vi "获取参数解析.vi"(11 "输入字符串":string) -> (3 "获取参数(定点数)":T1)   [LabVIEW 2016, in "环境动力监测库.lvlib" / "空调库.lvlib"]
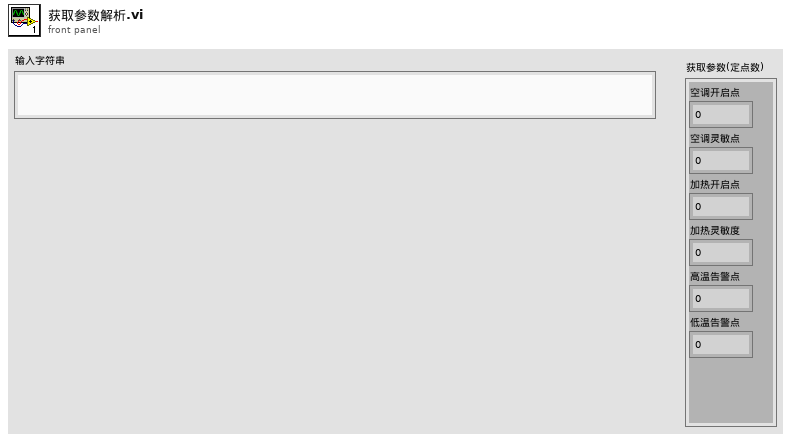
[diagram p1: front panel]
types:
  T1 = cluster{"空调开启点":u16, "空调灵敏点":u16, "加热开启点":u16, "加热灵敏度":u16, "高温告警点":u16, "低温告警点":u16}
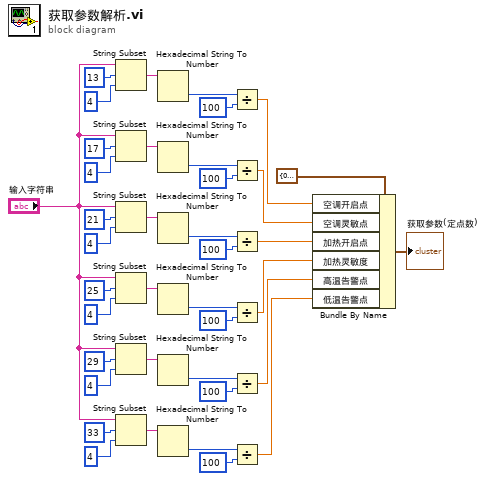
[diagram p0: block diagram]
diagram:
  n1 = String Subset(string="输入字符串", offset (0)=13 ("偏移量(0)"), length (rest)=4 ("长度（剩余）")) -> (substring=w37:string)
  n2 = String Subset(string="输入字符串", offset (0)=17 ("偏移量(0)"), length (rest)=4 ("长度（剩余）")) -> (substring=w34:string)
  n3 = String Subset(string="输入字符串", offset (0)=21 ("偏移量(0)"), length (rest)=4 ("长度（剩余）")) -> (substring=w33:string)
  n4 = String Subset(string="输入字符串", offset (0)=25 ("偏移量(0)"), length (rest)=4 ("长度（剩余）")) -> (substring=w28:string)
  n5 = String Subset(string="输入字符串", offset (0)=29 ("偏移量(0)"), length (rest)=4 ("长度（剩余）")) -> (substring=w20:string)
  n6 = String Subset(string="输入字符串", offset (0)=33 ("偏移量(0)"), length (rest)=4 ("长度（剩余）")) -> (substring=w25:string)
  n7 = Hexadecimal String To Number(string=w37) -> (number=w18:u32)  [unwired: 2 in, 1 out]
  n8 = Hexadecimal String To Number(string=w34) -> (number=w14:u32)  [unwired: 2 in, 1 out]
  n9 = Hexadecimal String To Number(string=w33) -> (number=w9:u32)  [unwired: 2 in, 1 out]
  n10 = Hexadecimal String To Number(string=w28) -> (number=w7:u32)  [unwired: 2 in, 1 out]
  n11 = Hexadecimal String To Number(string=w20) -> (number=w6:u32)  [unwired: 2 in, 1 out]
  n12 = Hexadecimal String To Number(string=w25) -> (number=w2:u32)  [unwired: 2 in, 1 out]
  n13 = Divide(x=w18, y=u32 100) -> (x/y=w16:dbl)
  n14 = Divide(x=w14, y=u32 100) -> (x/y=w13:dbl)
  n15 = Divide(x=w9, y=u32 100) -> (x/y=w8:dbl)
  n16 = Divide(x=w7, y=u32 100) -> (x/y=w5:dbl)
  n17 = Divide(x=w6, y=u32 100) -> (x/y=w4:dbl)
  n18 = Divide(x=w2, y=u32 100) -> (x/y=w1:dbl)
  n19 = Bundle By Name(cluster=T1 {"空调开启点"=0, "空调灵敏点"=0, "加热开启点"=0, "加热灵敏度"=0, "高温告警点"=0, "低温告警点"=0} ("获取参数(定点数)"), "空调开启点"=w16, "空调灵敏点"=w13, "加热开启点"=w8, "加热灵敏度"=w5, "高温告警点"=w4, "低温告警点"=w1) -> (→"获取参数(定点数)":T1)
